vi "DFD Integer Delay (Array).vi"(7 "init? (F)":bool, 8 "error in (no error)":errorcluster, 10 "delay":i32, 11 "signal in":dbl[](array[numeric])) -> (0 "error out":errorcluster, 3 "signal out":dbl[](array[numeric]))   [LabVIEW 2017, in "NI_DigFilterLicensed.lvlib"]
doc: "Delays a signal continuously by a specified integer number of sample intervals. Wire data to the <B>signal in</B> input to determine the polymorphic instance to use or manually select the instance."
uses:
  <vilib>/addons/Digital Filter Design/NI_DigFilterLicensed.lvlib
  <vilib>/addons/Digital Filter Design/Process.llb/DFD Integer Delay with State (Array).vi
  <vilib>/addons/Digital Filter Design/NI_DigFilter_Process.lvlib
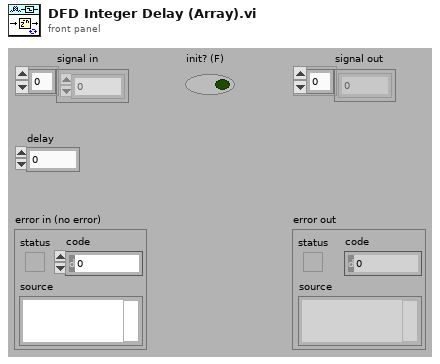
[diagram p1: front panel]
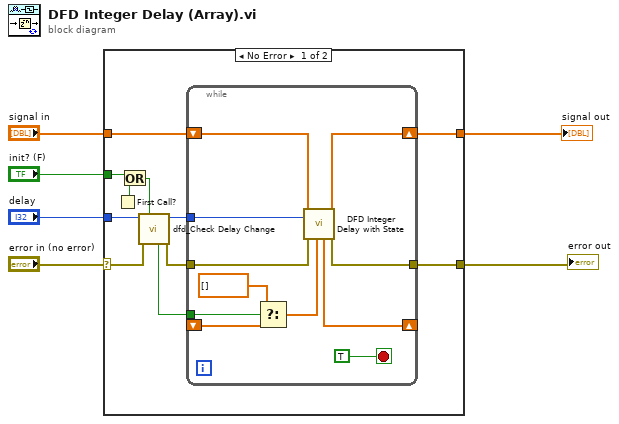
[diagram p0: block diagram]
diagram:
  n1 = case shown="No Error" "error in (no error)" {
    selector: "error in (no error)" -> [w10 w29]
    tunnel: [w15 w29] -> w5
    tunnel: "signal in" -> [w17 _]
    tunnel: [w16 _] -> w3
    tunnel: "delay" -> [w12 _]
    tunnel: "init? (F)" -> [w13 _]
    frame No Error {
      n2 = First Call?() -> (First Call?: T/F=w14:bool)
      n3 = Or(x=w13, y=w14) -> (x .or. y?=w8:bool)
      n4 = call <vilib>:"dfd_Check Delay Change.vi"("init in"=w8, "error in (no error)"=w10, "delay in"=w12) -> ("error out"=w7:errorcluster, "delay out"=w11:i32, "init out"=w9:bool)  [unwired: 6 out]
      n5 = while {
        shift-right: [w21] -> _
        shift-left: _ -> [w27]
        tunnel: [w18] -> w15
        tunnel: w9 -> [w25]
        tunnel: w11 -> [w26]
        shift-right: [w23] -> w16
        shift-left: w17 -> [w22]
        tunnel: w7 -> [w19]
        stop <- TRUE stop-if-true
        n6 = Select(t=dbl[] [], s=w25, f=w27) -> (s? t:f=w20:dbl[])
        n7 = call-poly <vilib>:"DFD Integer Delay with State.vi"("state in"=w20, "error in (no error)"=w19, "delay"=w26, "signal in"=w22) -> ("error out"=w18:errorcluster, "signal out"=w23:dbl[], "state out"=w21:dbl[])  [unwired: 5 out]
      }
    }
    frame Error {
    }
  }
  "error out" <- w5
  "signal out" <- w3
